vi "Main.vi"(10 "SP_Analisis":refnum<vi>, 11 "Module Admin":refnum<class "Delacor_lib_QMH_Module Admin.lvclass">) -> ()   [LabVIEW 2019, in "Analisis.lvlib"]
doc: "This template is based off of the Queued Message Handler design pattern and the Queued Message Handler project template that ships with LabVIEW.\n\nThe main difference is that the queue is private to this module and communication between modules is performed via Broadcast and Request events.\n\nRequest events are wrapped in public API methods and are handled in the Event Handling Loop (EHL) of this VI. Any module can register for Broadcast events sent by this module. The EHL generates messages based on user interface actions.\n\nThe Message Handling Loop (MHL) processes messages generated by the EHL, or by other messages. The messages are string values, so new messages can be added easily to the Message Cases case structure in the MHL. Each message cluster can also provide an optional value for Message Data, which is a variant that can be converted to whatever message-specific data is required.\n_____\nBased on Delacor QMH Project Template 5.0.0.82."
uses:
  Analisis.lvlib
  <vilib>/Delacor/Delacor QMH/Libraries/Module Admin_class/Delacor_lib_QMH_Module Admin.lvclass
  Module Data--cluster.ctl
  Stop Argument--cluster.ctl
  <vilib>/Delacor/Delacor QMH/Libraries/Message Queue_class/Delacor_lib_QMH_Message Queue.lvclass/Delacor_lib_QMH_Message Queue.ctl
  <vilib>/Delacor/Delacor QMH/Libraries/Module Admin_class/Delacor_lib_QMH_Module Admin.lvclass/Delacor_lib_QMH_Module Admin.ctl
  Analize and Conert Data Argument--cluster.ctl
  Aquiere the delay time configurated Argument--cluster.ctl
  <vilib>/Utility/miscctls.llb/LVPointTypeDef.ctl
  <vilib>/Delacor/Delacor QMH/Libraries/Message Queue_class/Delacor_lib_QMH_Enqueue Message (Single).vi
  <vilib>/Delacor/Delacor QMH/Libraries/Module Admin_class/Delacor_lib_QMH_Get External Launch.vi
  <vilib>/Utility/error.llb/Error Cluster From Error Code.vi
  <vilib>/ErrorRing/Error Ring.xnode
  <vilib>/Delacor/Delacor QMH/Libraries/Message Queue_class/Delacor_lib_QMH_Message Queue.lvclass
  Save DB_SQLite/Save DB_SQLite.lvlib
panel:
  out "Temperatura  °C":dbl(graph)
  out "Humedad       %":dbl(graph)
  out "Corriente":dbl
  out "Resistencia":i32
  out "Voltaje":dbl
  out "error out":errorcluster
  out "Status":string
  # "Entrada Analógica"
  # "%"
  # "Volts"
  # "Amperes"
  # "°C"
  # "Ohms"
  # "RICH TECH."
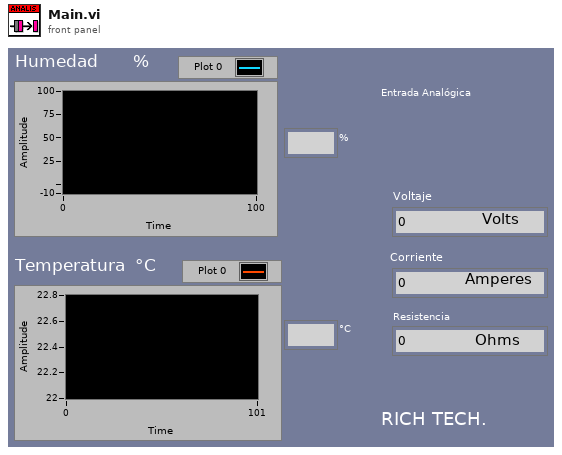
[diagram p1: front panel]
types:
  T1 = typedef "Analisis.lvlib/Request Events--cluster.ctl" = cluster{"Stop Module":refnum<user-event>, "Show Panel":refnum<user-event>, "Hide Panel":refnum<user-event>, "Get Module Execution Status":refnum<user-event>, "Show Diagram":refnum<user-event>, "Analize and Conert Data":refnum<user-event>, "Aquiere the delay time configurated":refnum<user-event>}
  T2 = typedef "Analisis.lvlib/Module Data--cluster.ctl" = cluster{"Status":string, "Time":i32}
  T3 = enum32{"invalid lock state", "Not Locked", "Locked (No Password)", "Password-protected"}
  T4 = typedef "Analisis.lvlib/Stop Argument--cluster.ctl" = cluster{"Origin":string, "Exit via Stop Module Req?":bool, "Wait for Module to stop?":bool}
  T5 = typedef "Analisis.lvlib/Analize and Conert Data Argument--cluster.ctl" = cluster{"Data":string}
  T6 = typedef "Analisis.lvlib/Aquiere the delay time configurated Argument--cluster.ctl" = cluster{"Time":i32}
  T7 = typedef "LVPointTypeDef.ctl" = cluster{"Horizontal":i16, "Vertical":i16}
  T8 = enum32{"Invalid", "Standard", "Closed", "Hidden", "Minimized", "Maximized"}
  T9 = cluster{"Humedad":dbl, "Temperatura":dbl, "Voltaje":dbl, "Corriente":dbl, "Resistencia":i32}
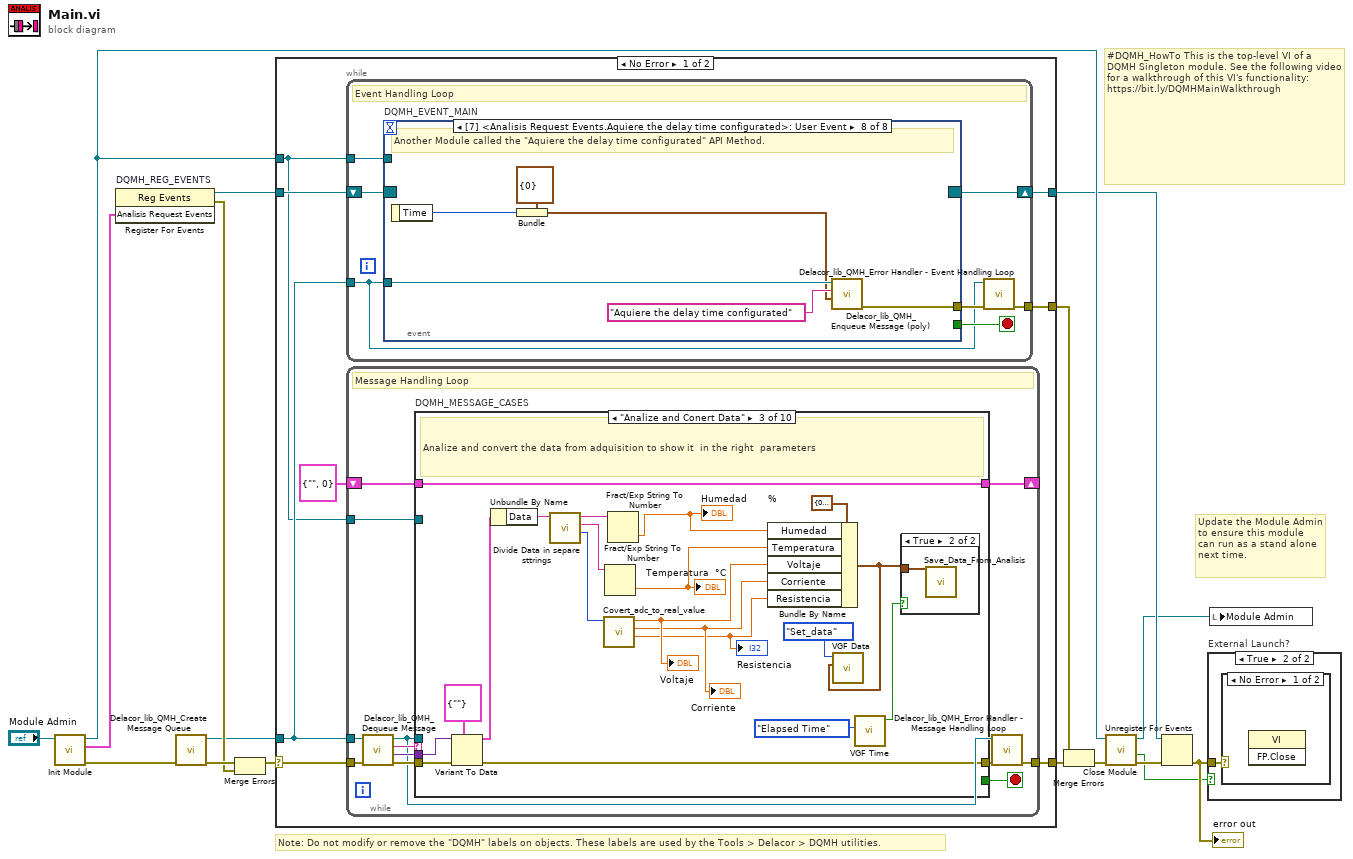
[diagram p0: block diagram]
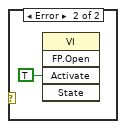
[diagram p3: hidden frame]
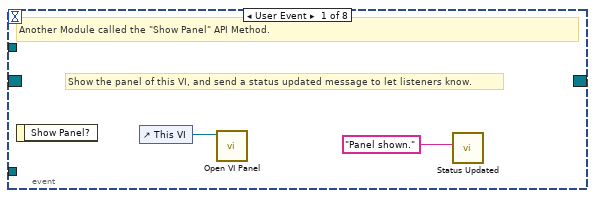
[diagram p4: hidden frame]
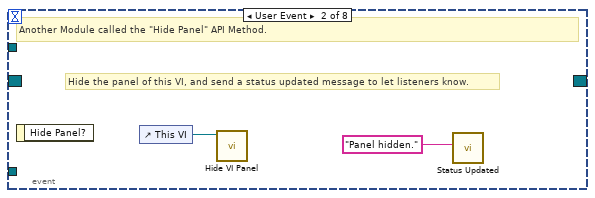
[diagram p5: hidden frame]
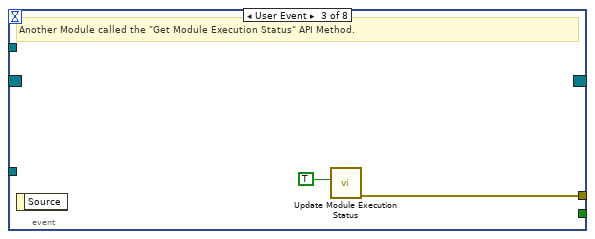
[diagram p6: hidden frame]
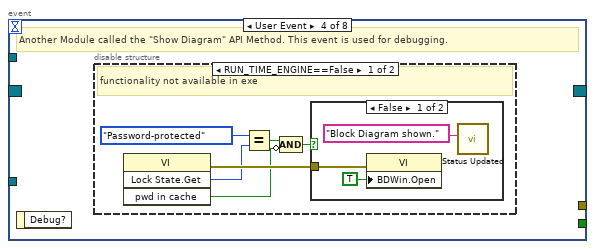
[diagram p7: hidden frame]
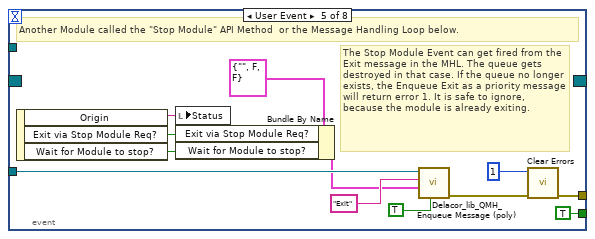
[diagram p10: hidden frame]
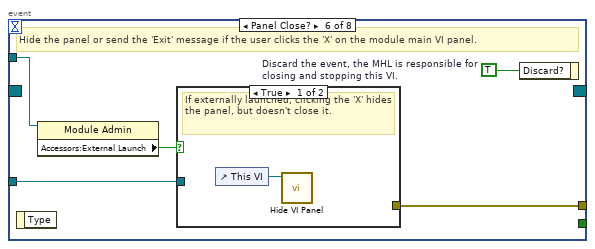
[diagram p11: hidden frame]
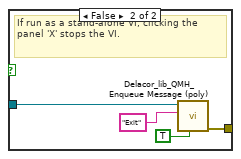
[diagram p12: hidden frame]
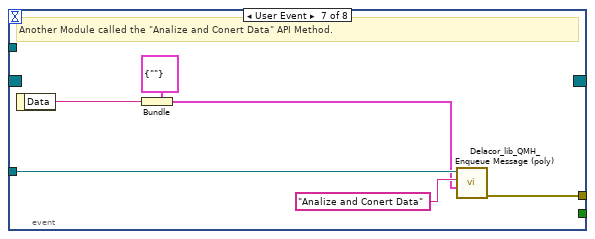
[diagram p13: hidden frame]
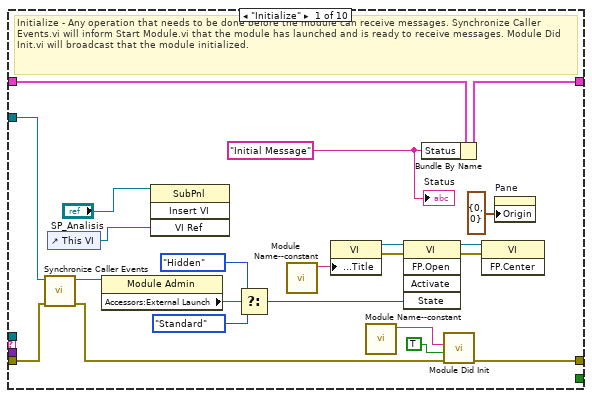
[diagram p14: hidden frame]
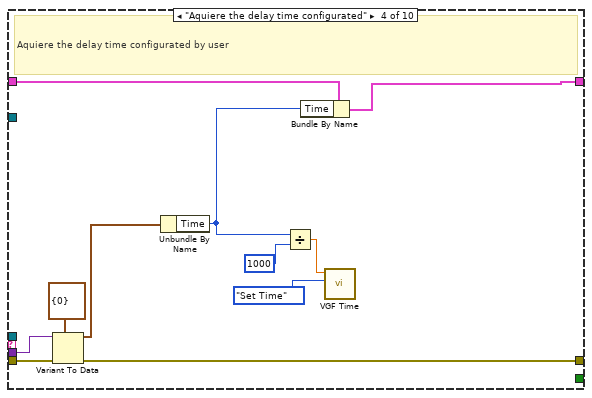
[diagram p17: hidden frame]
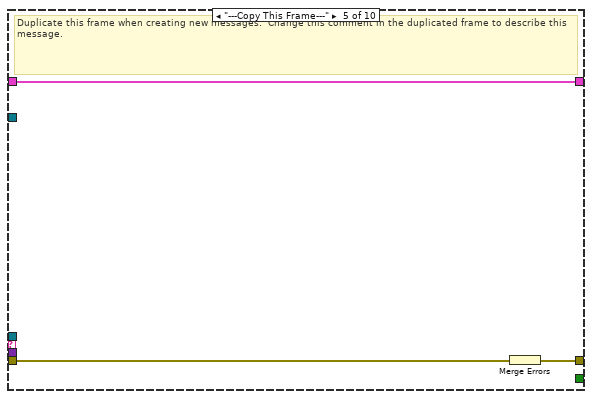
[diagram p18: hidden frame]
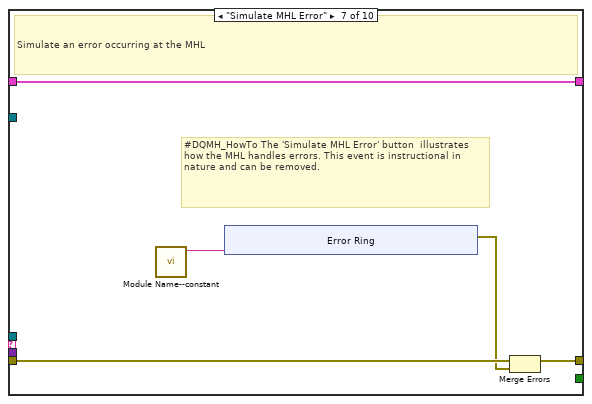
[diagram p20: hidden frame]
diagram:
  # "#DQMH_HowTo This is the top-level VI of a DQMH Singleton module. See the following video for a walkthrough of this VI's functionality: https://bit.ly/DQMHMainWalkthrough"
  # "Note: Do not modify or remove the \"DQMH\" labels on objects. These labels are used by the Tools > Delacor > DQMH utilities."
  # "Update the Module Admin to ensure this module can run as a stand alone next time."
  n1 = call "Init Module.vi"("Singleton Module Admin in"="Module Admin") -> ("error out"=w16:errorcluster, "Analisis Request Events"=w5:T1, "Singleton Module Admin out"=w8:refnum<class "Delacor_lib_QMH_Module Admin.lvclass">)  [unwired: 8 in]
  n2 = register-events "DQMH_REG_EVENTS"(w5) -> (reference out=w6:refnum<event-registration>, error out=w9:errorcluster)  [unwired: 2 in]
  n3 = call <vilib>:"Delacor_lib_QMH_Create Message Queue.vi"("error in (no error)"=w16) -> ("error out"=w11:errorcluster, "Message Queue"=w4:refnum<class "Delacor_lib_QMH_Message Queue.lvclass">)  [unwired: 9 in]
  n4 = Merge Errors(w11, w9) -> (w10:errorcluster)
  n5 = case shown="No Error" w10 {
    selector: w10 -> [w23 w215]
    tunnel: [w25 w214] -> w17
    tunnel: [w22 w220] -> w7
    tunnel: w6 -> [w20 w220]
    tunnel: w4 -> [w19 w213]
    tunnel: [w24 _] -> w14
    tunnel: w8 -> [w18 w216]
    frame No Error {
      n6 = while {
        tunnel: w19 -> [w26]
        shift-right: [w29] -> w22
        shift-left: w20 -> [w30]
        tunnel: [w31] -> w24
        tunnel: w18 -> [w27]
        stop <- w28 stop-if-true
        # "Event Handling Loop"
        n7 = event "DQMH_EVENT_MAIN" shown="[7] <Analisis Request Events.Aquiere the delay time configurated>: User Event" {
          selector: w30 -> [_ _ _ _ _ _ _ _]
          dyn-events: [_ _ _ _ _ _ _ _] -> w29
          timeout: _ -> [_ _ _ _ _ _ _ _]
          tunnel: [_ _ _ _ TRUE ("Discard?") _ _ _] -> w28
          tunnel: w26 -> [_ _ _ _ w55 w62 w75 w81]
          tunnel: [_ _ w38 _ w58 w64 w70 w76] -> w32
          tunnel: w27 -> [_ _ _ _ _ w61 _ _]
          event User Event {
            # "Show the panel of this VI, and send a status updated message to let listeners know."
            # "Another Module called the \"Show Panel\" API Method."
            n8 = event-data() -> ()  [unwired: 1 in, 1 out]
            n9 = control-ref of="This VI"() -> (w34:refnum<vi>)
            n10 = call "Open VI Panel.vi"("VI"=w34) -> ()  [unwired: 10 in, 1 out]
            n11 = call "Status Updated.vi"("Status"="Panel shown." ("format string")) -> ()  [unwired: 10 in, 1 out]
          }
          event User Event {
            # "Hide the panel of this VI, and send a status updated message to let listeners know."
            # "Another Module called the \"Hide Panel\" API Method."
            n12 = event-data() -> ()  [unwired: 1 in, 1 out]
            n13 = control-ref of="This VI"() -> (w36:refnum<vi>)
            n14 = call "Hide VI Panel.vi"("VI"=w36) -> ()  [unwired: 10 in, 1 out]
            n15 = call "Status Updated.vi"("Status"="Panel hidden." ("format string")) -> ()  [unwired: 10 in, 1 out]
          }
          event User Event {
            # "Another Module called the \"Get Module Execution Status\" API Method."
            n16 = event-data() -> ()  [unwired: 1 in, 1 out]
            n17 = call "Update Module Execution Status.vi"("Running?"=TRUE) -> ("error out"=w38:errorcluster)  [unwired: 10 in]
          }
          event User Event {
            # "Another Module called the \"Show Diagram\" API Method. This event is used for debugging."
            n18 = event-data() -> ()  [unwired: 1 in, 1 out]
            n19 = disable-structure shown="RUN_TIME_ENGINE==False" {
              frame condition #0 (active) {
                # "functionality not available in exe"
                n20 = invoke class="VI" method="Lock State.Get"() -> (error out=w44:errorcluster, "Get Lock State"=w43:T3, "pwd in cache"=w40:bool)  [unwired: 4 in, 1 out]
                n21 = Equal?(x=T3."Password-protected", y=w43) -> (x = y?=w41:bool)
                n22 = Compound Arithmetic op=AND(w41, invert w40) -> (w39:bool)
                n23 = case shown="False" w39 {
                  tunnel: w44 -> [w47 _]
                  frame False {
                    n24 = property class="VI"(error in=w47, "BDWin.Open"=TRUE ("Block Diagram Window:Open")) -> ()  [unwired: 1 in, 2 out]
                    n25 = call "Status Updated.vi"("Status"="Block Diagram shown." ("format string")) -> ()  [unwired: 10 in, 1 out]
                  }
                  frame True {
                    # "Password-protected VI, and the password is not in the cache. Do not show the diagram."
                  }
                }
              }
              frame condition #1 {
              }
            }
          }
          event User Event {
            # "The Stop Module Event can get fired from the Exit message in the MHL. The queue gets destroyed in that case. If the queue no longer exists, the Enqueue Exit as a priority message will return error 1. It is safe to ignore, because the module is already exiting."
            # "Another Module called the \"Stop Module\" API Method  or the Message Handling Loop below."
            n26 = event-data() -> ("Origin"=w54:string, "Exit via Stop Module Req?"=w50:bool, "Wait for Module to stop?"=w49:bool)  [unwired: 1 in]
            n27 = local write "Status"(w54) -> ()
            n28 = Bundle By Name(cluster=T4 {"Origin"="", "Exit via Stop Module Req?"=FALSE, "Wait for Module to stop?"=FALSE} ("Stop Argument"), "Exit via Stop Module Req?"=w50, "Wait for Module to stop?"=w49) -> (w48:T4)
            n29 = call-poly <vilib>:"Delacor_lib_QMH_Enqueue Message (poly).vi"("Priority Message? (F)"=TRUE, "Message Data"=w48, "Message"="Exit", "Message Queue in"=w55) -> ("error out"=w59:errorcluster)  [unwired: 6 in, 1 out]
            n30 = call <vilib>:"Clear Errors.vi"("error in (no error)"=w59, "specific error code to clear (0: all)"=1) -> ("error out"=w58:errorcluster)  [unwired: 4 in, 1 out]
          }
          event Panel Close? {
            w63 = TRUE  # Discard the event, the MHL is responsible for closing and stopping this VI.
            # "Hide the panel or send the 'Exit' message if the user clicks the 'X' on the module main VI panel."
            n31 = event-data() -> ()  [unwired: 1 in, 1 out]
            n32 = property class="Module Admin"(reference=w61) -> ("Accessors:External Launch"=w60:bool)  [unwired: 1 in, 2 out]
            n33 = case shown="True" w60 {
              tunnel: w62 -> [_ w68]
              tunnel: [_ w69] -> w64
              frame True {
                # "If externally launched, clicking the 'X' hides the panel, but doesn't close it."
                n34 = control-ref of="This VI"() -> (w65:refnum<vi>)
                n35 = call "Hide VI Panel.vi"("VI"=w65) -> ()  [unwired: 10 in, 1 out]
              }
              frame False {
                # "If run as a stand-alone VI, clicking the panel 'X' stops the VI."
                n36 = call-poly <vilib>:"Delacor_lib_QMH_Enqueue Message (poly).vi"("Priority Message? (F)"=TRUE, "Message"="Exit", "Message Queue in"=w68) -> ("error out"=w69:errorcluster)  [unwired: 7 in, 1 out]
              }
            }
            n37 = event-data("Discard?"=w63) -> ()  [unwired: 1 in, 1 out]
          }
          event User Event {
            # "Another Module called the \"Analize and Conert Data\" API Method."
            n38 = event-data() -> ("Data"=w71:string)  [unwired: 1 in]
            n39 = Bundle(cluster=T5 {"Data"=""} ("Analize and Conert Data Argument"), "Data"=w71) -> (w72:T5)
            n40 = call-poly <vilib>:"Delacor_lib_QMH_Enqueue Message (poly).vi"("Message Data"=w72, "Message"="Analize and Conert Data", "Message Queue in"=w75) -> ("error out"=w70:errorcluster)  [unwired: 7 in, 1 out]
          }
          event User Event {
            # "Another Module called the \"Aquiere the delay time configurated\" API Method."
            n41 = event-data() -> ("Time"=w77:u32)  [unwired: 1 in]
            n42 = Bundle(cluster=T6 {"Time"=0} ("Aquiere the delay time configurated Argument"), "Time"=w77) -> (w78:T6)
            n43 = call-poly <vilib>:"Delacor_lib_QMH_Enqueue Message (poly).vi"("Message Data"=w78, "Message"="Aquiere the delay time configurated", "Message Queue in"=w81) -> ("error out"=w76:errorcluster)  [unwired: 7 in, 1 out]
          }
        }
        n44 = call-dynamic "Delacor_lib_QMH_Error Handler - Event Handling Loop.vi"("error in (no error)"=w32, "Message Queue in"=w26) -> ("dup error in"=w31:errorcluster)  [unwired: 8 in, 1 out]
      }
      n45 = while {
        tunnel: w19 -> [w84]
        shift-right: [w88] -> _
        shift-left: T2 {"Status"="", "Time"=0} ("Data Cluster") -> [w89]
        tunnel: w23 -> [w92]
        tunnel: [w90] -> w25
        tunnel: w18 -> [w82]
        stop <- w87 stop-if-true
        # "Message Handling Loop"
        n46 = call-dynamic "Delacor_lib_QMH_Dequeue Message.vi"("error in (no error)"=w92, "Message Queue in"=w84) -> ("error out"=w91:errorcluster, "Message Data"=w85:variant, "Message"=w86:string, "Message Queue out"=w83:refnum<class "Delacor_lib_QMH_Message Queue.lvclass">)  [unwired: 6 in]
        n47 = case "DQMH_MESSAGE_CASES" shown="\"Analize and Conert Data\"" w86 {
          selector: w86 -> [_ _ _ _ _ _ _ _ _ w200]
          tunnel: w83 -> [_ _ _ _ _ _ _ w170 w192 _]
          tunnel: w91 -> [w113 w117 w137 w149 w152 w154 w159 w177 w198 w202]
          tunnel: [w111 w117 w136 w148 w151 w154 w158 w173 w195 w203] -> w93
          tunnel: w89 -> [w102 w116 w127 w144 w150 w153 w156 w172 w191 w201]
          tunnel: [w101 w116 w127 w143 w150 w153 w156 w172 w191 w201] -> w88
          tunnel: [_ _ _ _ _ _ _ _ w190 _] -> w87
          tunnel: w85 -> [_ _ w135 w147 _ _ _ w171 w189 _]
          tunnel: w82 -> [w103 _ _ _ _ _ _ w169 w184 _]
          frame "Initialize" {
            w96 = "Initial Message" ("Initial Message")
            # "Initialize - Any operation that needs to be done before the module can receive messages. Synchronize Caller Events.vi will inform Start Module.vi that the module has launched and is ready to receive messages. Module Did Init.vi will broadcast that the module initialized."
            n48 = call "Synchronize Caller Events.vi"("error in (no error)"=w113, "Singleton Module Admin in"=w103) -> ("error out"=w112:errorcluster, "Singleton Module Admin out"=w98:refnum<class "Delacor_lib_QMH_Module Admin.lvclass">)  [unwired: 8 in]
            n49 = control-ref of="This VI"() -> (w95:refnum<vi>)
            n50 = property class="Module Admin"(reference=w98) -> ("Accessors:External Launch"=w107:bool)  [unwired: 1 in, 2 out]
            n51 = invoke class="SubPnl" method="Insert VI"(reference="SP_Analisis", "VI Ref"=w95) -> ()  [unwired: 2 in, 4 out]
            n52 = Select(t=T8."Hidden" ("State"), s=w107, f=T8."Standard" ("State")) -> (s? t:f=w104:T8)
            n53 = call "Module Name--constant.vi"() -> ("Module Name"=w110:string)  [unwired: 11 in]
            n54 = property class="VI"("Front Panel.Title"=w110) -> (reference out=w109:refnum<vi>, error out=w115:errorcluster)  [unwired: 2 in]
            n55 = call "Module Name--constant.vi"() -> ("Module Name"=w99:string)  [unwired: 11 in]
            n56 = invoke class="VI" method="FP.Open"(reference=w109, error in=w115, "State"=w104) -> (reference out=w108:refnum<vi>, error out=w114:errorcluster)  [unwired: 2 in, 3 out]
            n57 = Bundle By Name(cluster=w102, "Status"=w96) -> (w101:T2)
            n58 = call "Module Did Init.vi"("error in (no error)"=w112, "Initialized?"=TRUE, "Origin"=w99) -> ("error out"=w111:errorcluster)  [unwired: 8 in]
            n59 = invoke class="VI" method="FP.Center"(reference=w108, error in=w114) -> ()  [unwired: 1 in, 3 out]
            n60 = property on="Pane" class="Pane"("Origin"=T7 {"Horizontal"=0, "Vertical"=0}) -> ()  [unwired: 2 in, 2 out]
            "Status" <- w96
          }
          frame "--- Module Specific ---" {
            # "Separator -- The following cases handle messages specific to this Module."
          }
          frame "Analize and Conert Data" {
            # "Analize and convert the data from adquisition to show it  in the right  parameters"
            n61 = Variant To Data(error in=w137, type=T5 {"Data"=""} ("Analize and Conert Data Argument"), Variant=w135) -> (data=w133:T5, error out=w136:errorcluster)
            n62 = Unbundle By Name(w133) -> ("Data"=w132:string)
            n63 = call "Divide Data in separe sttrings.vi"("Data"=w132) -> ("ADC"=w131:i32, "Temperatura"=w130:string, "Humedad"=w129:string)  [unwired: 8 in]
            n64 = call "Covert_adc_to_real_value.vi"("ADC"=w131) -> ("Resistencia"=w118:dbl, "Corriente"=w119:dbl, "Voltaje"=w120:dbl)  [unwired: 8 in]
            "Voltaje" <- w120
            "Resistencia" <- w118
            "Corriente" <- w119
            n65 = Fract/Exp String To Number(string=w130) -> (number=w125:dbl)  [unwired: 3 in, 1 out]
            "Temperatura  °C" <- w125
            n66 = Fract/Exp String To Number(string=w129) -> (number=w126:dbl)  [unwired: 3 in, 1 out]
            "Humedad       %" <- w126
            n67 = Bundle By Name(cluster=T9 {"Humedad"=0.0, "Temperatura"=0.0, "Voltaje"=0.0, "Corriente"=0.0, "Resistencia"=0} ("Data"), "Humedad"=w126, "Temperatura"=w125, "Voltaje"=w120, "Corriente"=w119, "Resistencia"=w118) -> (w121:T9)
            n68 = call "VGF Data.vi"("Data"=w121, "Accion"=enum16{"Read", "Set_data"}."Set_data") -> ()  [unwired: 9 in, 1 out]
            n69 = call "VGF Time.vi"("Enum"=enum16{"Set Time", "Elapsed Time"}."Elapsed Time") -> ("Time lapsed"=w123:bool)  [unwired: 10 in]
            n70 = case shown="True" w123 {
              tunnel: w121 -> [_ w138]
              frame False {
              }
              frame True {
                n71 = call "Save_Data_From_Analisis.vi"("Data"=w138) -> ()  [unwired: 10 in, 1 out]
              }
            }
          }
          frame "Aquiere the delay time configurated" {
            # "Aquiere the delay time configurated by user"
            n72 = Variant To Data(error in=w149, type=T6 {"Time"=0} ("Aquiere the delay time configurated Argument"), Variant=w147) -> (data=w145:T6, error out=w148:errorcluster)
            n73 = Unbundle By Name(w145) -> ("Time"=w139:i32)
            n74 = Divide(x=w139, y=1000) -> (x/y=w140:dbl)
            n75 = Bundle By Name(cluster=w144, "Time"=w139) -> (w143:T2)
            n76 = call "VGF Time.vi"("Enum"=enum16{"Set Time", "Elapsed Time"}."Set Time", "Time tarjet"=w140) -> ()  [unwired: 9 in, 1 out]
          }
          frame "---Copy This Frame---" {
            # "Duplicate this frame when creating new messages.  Change this comment in the duplicated frame to describe this message."
            n77 = Merge Errors(w152) -> (w151:errorcluster)
          }
          frame "--- Exit and Error Handling---" {
            # "Separator - The following cases handle errors and exit messages."
          }
          frame "Simulate MHL Error" {
            # "#DQMH_HowTo The 'Simulate MHL Error' button  illustrates how the MHL handles errors. This event is instructional in nature and can be removed."
            # "Simulate an error occurring at the MHL"
            n78 = call "Module Name--constant.vi"() -> ("Module Name"=w155:string)  [unwired: 11 in]
            n79 = xnode "Error Ring"("parameter 0"=w155) -> ("error out"=w157:errorcluster)
            n80 = Merge Errors(w159, w157) -> (w158:errorcluster)
          }
          frame "Error" {
            # "#CodeRecommended - If you ever change the name of this \"Error\" message, you'll need to update the name in the Check Loop Error.vi as well."
            # "#CodeRecommended - If the module is running in standalone mode (External Launch = FALSE), this code will pop up an error dialog and call the 'Exit' message if an error occurs. Add more fine-grained error handling here."
            # "Error - Check the error message data and respond accordingly. This message is sent by the \"Error Handler\" VIs at the end of each loop in this application."
            n81 = property class="Module Admin"(reference=w169) -> ("Accessors:External Launch"=w168:bool)  [unwired: 1 in, 2 out]
            n82 = Variant To Data(error in=w177, type=errorcluster {"status"=FALSE, "code"=0, "source"=""} ("error constant"), Variant=w171) -> (data=w178:errorcluster, error out=w175:errorcluster)
            n83 = call "Module Name--constant.vi"() -> ("Module Name"=w167:string)  [unwired: 11 in]
            n84 = call "Error Reported.vi"("Additional Information"=w167, "Error"=w178) -> ()  [unwired: 9 in, 1 out]
            n85 = case shown="False" w168 {
              tunnel: [w183 _] -> w174
              tunnel: w170 -> [w181 _]
              tunnel: w178 -> [w182 _]
              frame False {
                # "If the module is running standalone, then pop up an error dialog and call the \"Exit\" message."
                n86 = call <vilib>:"Simple Error Handler.vi"("error in (no error)"=w182) -> ()  [unwired: 4 in, 5 out]
                n87 = call-poly <vilib>:"Delacor_lib_QMH_Enqueue Message (poly).vi"("Priority Message? (F)"=TRUE, "Message"="Exit", "Message Queue in"=w181) -> ("error out"=w183:errorcluster)  [unwired: 7 in, 1 out]
              }
              frame True {
                # "If the module was launched externally, calling the Error Reported broadcast VI is the only action performed by the \"Error\" message. The module's caller can then process the error appropriately."
              }
            }
            n88 = Merge Errors(w175, w174) -> (w173:errorcluster)
            n89 = local write "error out"(w173) -> ()
          }
          frame "Exit" {
            w188 = 91  # 91: not all Exit messages will have an argument
            w190 = TRUE  # Stop the VI
            # "Release the message queue reference"
            # "#CodeNeeded - Add any required cleanup code here"
            # "Exit - Exit the application."
            n90 = Variant To Data(error in=w198, type=T4 {"Origin"="", "Exit via Stop Module Req?"=FALSE, "Wait for Module to stop?"=FALSE} ("Stop Argument"), Variant=w189) -> (data=w186:T4, error out=w194:errorcluster)
            n91 = call <vilib>:"Clear Errors.vi"("error in (no error)"=w194, "specific error code to clear (0: all)"=w188) -> ("error out"=w197:errorcluster)  [unwired: 4 in, 1 out]
            n92 = control-ref of="This VI"() -> (w185:refnum<vi>)
            n93 = call-dynamic "Delacor_lib_QMH_Release Message Queue.vi"("error in (no error)"=w197, "Message Queue"=w192) -> ("error out"=w196:errorcluster)  [unwired: 9 in]
            n94 = call "Handle Exit.vi"("Stop Argument"=w186, "Admin in"=w184, "VI reference"=w185) -> ("error out"=w193:errorcluster)  [unwired: 7 in, 1 out]
            n95 = Merge Errors(w196, w193) -> (w195:errorcluster)
          }
          frame Default {
            # "'Default' case only runs if there is a message that isn't defined in any of the other cases.  Output a programming error."
            n96 = call "Module Name--constant.vi"() -> ("Module Name"=w199:string)  [unwired: 11 in]
            n97 = xnode "Error Ring"("parameter 0"=w200, "parameter 1"=w199) -> ("error out"=w204:errorcluster)
            n98 = Merge Errors(w202, w204) -> (w203:errorcluster)
          }
        }
        n99 = call-dynamic "Delacor_lib_QMH_Error Handler - Message Handling Loop.vi"("error in (no error)"=w93, "Message Queue in"=w83) -> ("dup error in"=w90:errorcluster)  [unwired: 8 in, 1 out]
      }
    }
    frame Error {
      # "Synchronize Caller Events.vi will inform Start Module.vi that the module has launched and will let the code calling Start Module.vi register for broadcasts and would permit the caller receive the broadcast that an error occurred at launch time."
      n100 = call-dynamic "Delacor_lib_QMH_Release Message Queue.vi"("error in (no error)"=w215, "Message Queue"=w213) -> ("error out"=w214:errorcluster)  [unwired: 9 in]
      n101 = call "Synchronize Caller Events.vi"("Singleton Module Admin in"=w216) -> ("error out"=w221:errorcluster)  [unwired: 9 in, 1 out]
      n102 = call "Module Name--constant.vi"() -> ("Module Name"=w219:string)  [unwired: 11 in]
      n103 = Format Into String(format string="An error occurred during initialization. %s is no longer running.", w219) -> (resulting string=w217:string)  [unwired: 2 in, 1 out]
      n104 = Merge Errors(w214, w221) -> (w222:errorcluster)
      n105 = call "Error Reported.vi"("Additional Information"=w217, "Error"=w222) -> ()  [unwired: 9 in, 1 out]
    }
  }
  n106 = Merge Errors(w14, w17) -> (w13:errorcluster)
  n107 = call "Close Module.vi"("error in (no error)"=w13, "Module Admin in"=w8) -> ("error out"=w15:errorcluster, "External Launch"=w1:bool, "Module Admin out"=w2:refnum<class "Delacor_lib_QMH_Module Admin.lvclass">)  [unwired: 7 in]
  n108 = Unregister For Events(event registration refnum=w7, error in=w15) -> (error out=w12:errorcluster)
  "error out" <- w12
  n109 = case "External Launch?" shown="True" w1 {
    tunnel: w12 -> [_ w223]
    frame False {
    }
    frame True {
      n110 = case shown="No Error" w223 {
        frame No Error {
          n111 = invoke class="VI" method="FP.Close"() -> ()  [unwired: 3 in, 3 out]
        }
        frame Error {
          n112 = invoke class="VI" method="FP.Open"("Activate"=TRUE ("Activate?")) -> ()  [unwired: 4 in, 5 out]
        }
      }
    }
  }
  n113 = local write "Module Admin"(w2) -> ()
